vi "CC Restore Previous Setup.vi"() -> (2 "Select File":path, 3 "Restored?":bool)   [LabVIEW 2024]
panel:
  in  "Cancel":bool
  out "Contents":string
  in  "Restore":bool
  in  "Previous Setups":i32(listbox)
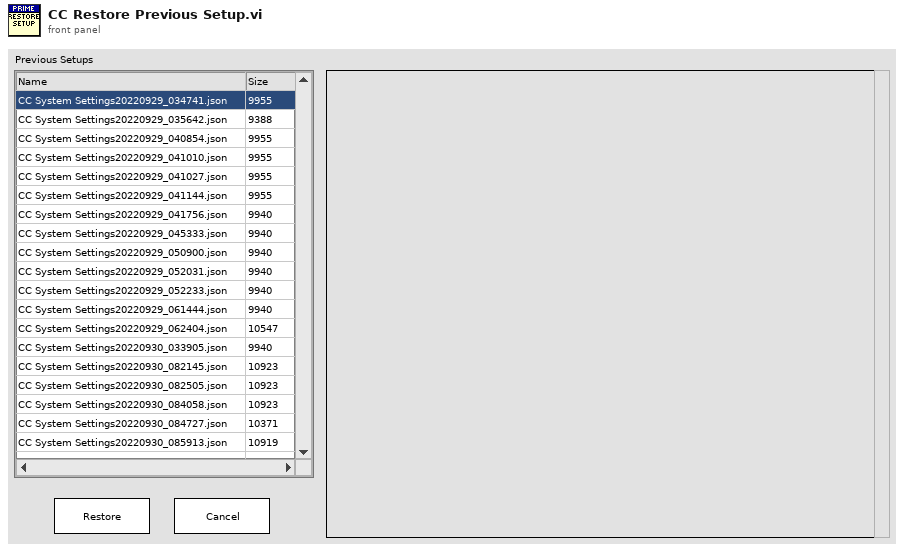
[diagram p1: front panel]
types:
  T1 = cluster{"state":refnum<user-event>, "Path":path, "Select File":path, "Restored?":bool}
  T2 = enum32{"invalid app kind", "Development System", "Run Time System", "Student Edition", "Embedded LabVIEW", "Evaluation", "Custom"}
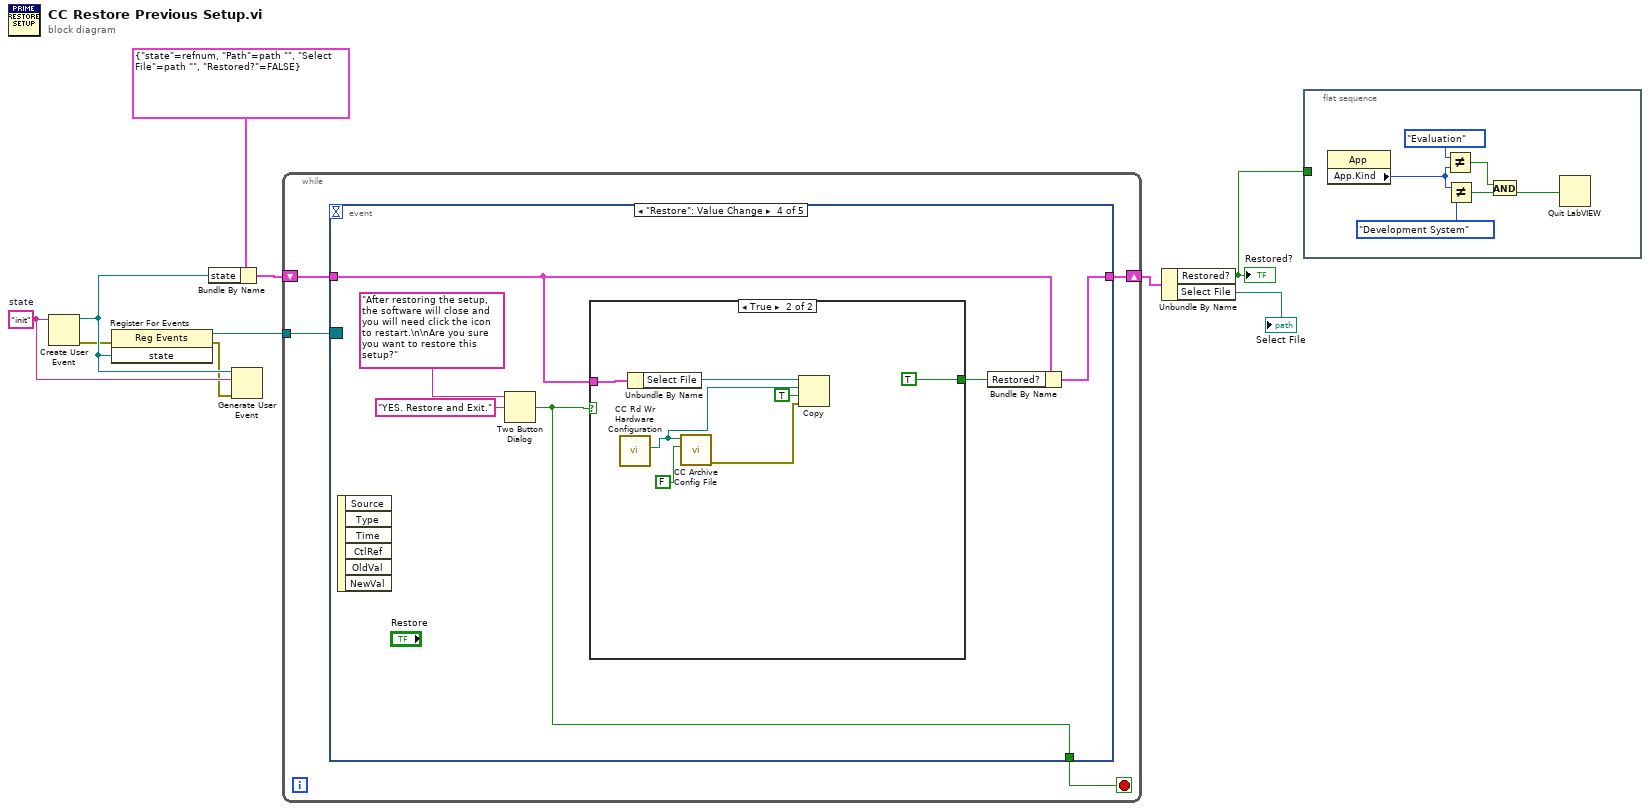
[diagram p0: block diagram]
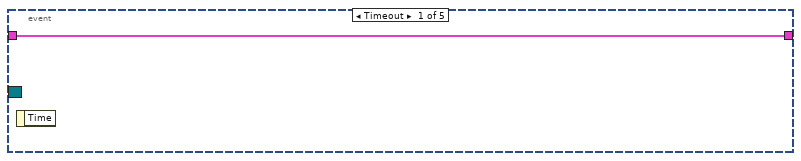
[diagram p2: hidden frame]
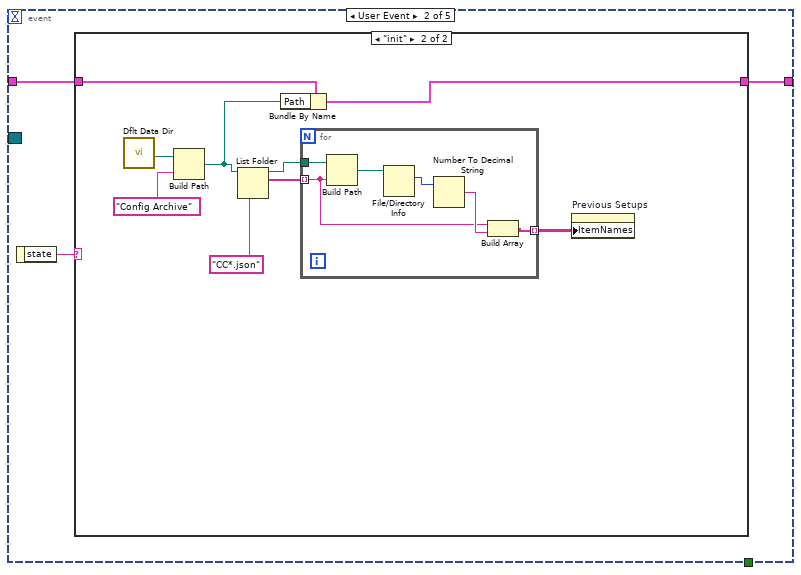
[diagram p3: hidden frame]
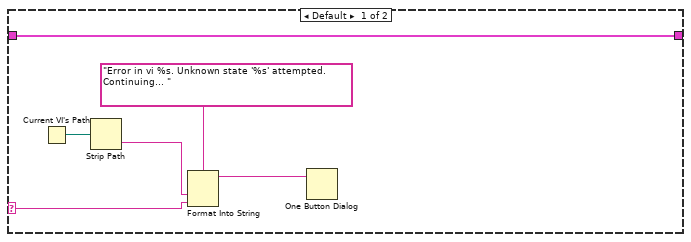
[diagram p4: hidden frame]
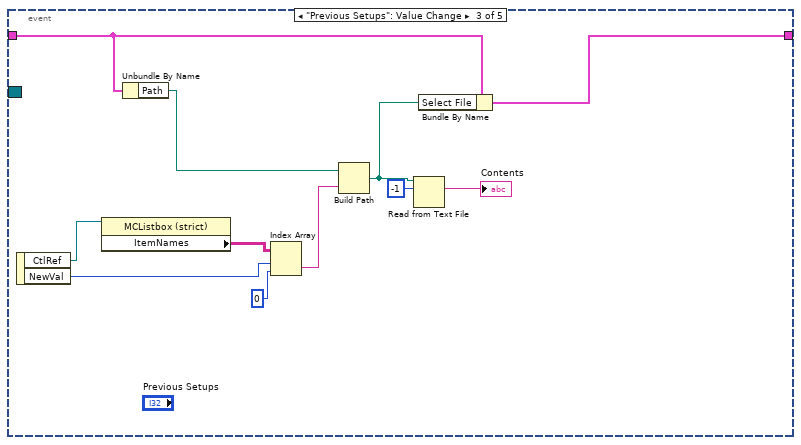
[diagram p5: hidden frame]
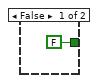
[diagram p6: hidden frame]
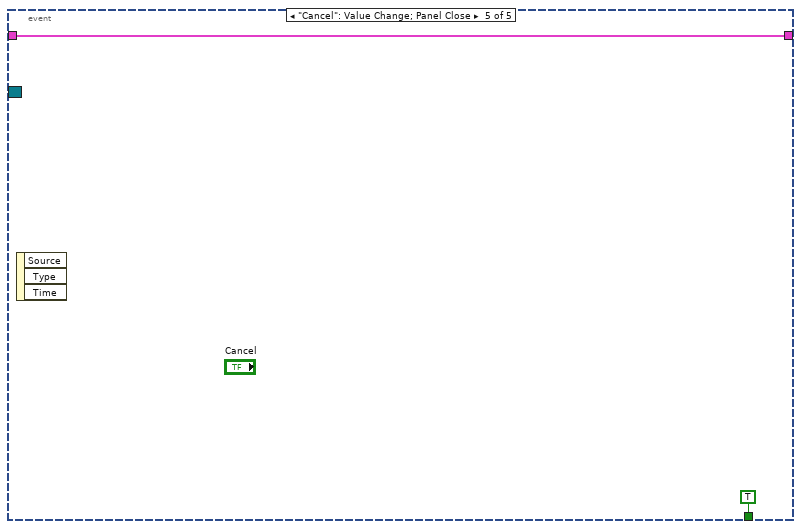
[diagram p7: hidden frame]
diagram:
  w6 = "init"  # state
  n1 = Create User Event(user event datatype=w6) -> (user event=w8:refnum<user-event>, error out=w4:errorcluster)  [unwired: 1 in]
  n2 = register-events(error in=w4, w8) -> (reference out=w7:refnum<event-registration>, error out=w5:errorcluster)  [unwired: 1 in]
  n3 = Bundle By Name(cluster=T1 {"state"=refnum, "Path"=path "", "Select File"=path "", "Restored?"=FALSE}, "state"=w8) -> (w9:T1)
  n4 = Generate User Event(user event=w8, event data cluster=w6, error in=w5) -> ()  [unwired: 1 in, 2 out]
  n5 = while {
    tunnel: w7 -> [w14]
    shift-right: [w12] -> w3
    shift-left: w9 -> [w13]
    stop <- w11 stop-if-true
    n6 = event shown="[3] \"Restore\": Value Change" {
      selector: w14 -> [_ _ _ _ _]
      dyn-events: _ -> [_ _ _ _ _]
      timeout: _ -> [_ _ _ _ _]
      tunnel: w13 -> [w15 w17 w40 w51 w66]
      tunnel: [w15 w16 w41 w52 w66] -> w12
      tunnel: [_ _ _ w54 TRUE ("Close")] -> w11
      event Timeout {
        n7 = event-data() -> ()  [unwired: 1 in, 1 out]
      }
      event User Event {
        n8 = event-data() -> ("state"=w18:string)  [unwired: 1 in]
        n9 = case shown="\"init\"" w18 {
          selector: w18 -> [w23 _]
          tunnel: w17 -> [w19 w25]
          tunnel: [w19 w26] -> w16
          frame Default {
            n10 = Current VI's Path() -> (path=w22:path)
            n11 = Strip Path(path=w22) -> (name=w21:string)  [unwired: 1 out]
            n12 = Format Into String(format string="Error in vi %s. Unknown state '%s' attempted. Continuing... ", w21, w23) -> (resulting string=w20:string)  [unwired: 2 in, 1 out]
            n13 = One Button Dialog(message=w20) -> ()  [unwired: 1 in, 1 out]
          }
          frame "init" {
            n14 = call <vilib>:"Dflt Data Dir.vi"() -> ("App:Default Data Directory"=w33:path)
            n15 = Build Path(base path=w33, name or relative path="Config Archive") -> (appended path=w27:path)
            n16 = List Folder(path=w27, pattern="CC*.json") -> (path out=w29:path, filenames=w30:string[])  [unwired: 2 in, 2 out]
            n17 = Bundle By Name(cluster=w25, "Path"=w27) -> (w26:T1)
            n18 = for {
              tunnel: w30 -> [w35] mode=indexing
              tunnel: w29 -> [w39]
              tunnel: [w34] -> w28 mode=indexing
              n19 = Build Path(base path=w39, name or relative path=w35) -> (appended path=w38:path)
              n20 = File/Directory Info(path=w38) -> (size=w37:i64)  [unwired: 1 in, 6 out]
              n21 = Number To Decimal String(number=w37) -> (decimal integer string=w36:string)  [unwired: 1 in]
              n22 = Build Array(w35, w36) -> (w34:string[])
            }
            n23 = property on="Previous Setups" class="MCListbox (strict)"("ItemNames"=w28) -> ()  [unwired: 2 in, 2 out]
          }
        }
      }
      event "Previous Setups": Value Change {
        n24 = event-data() -> ("CtlRef"=w50:refnum<vi>, "NewVal"=w48:i32)  [unwired: 1 in]
        n25 = property class="MCListbox (strict)"(reference=w50) -> ("ItemNames"=w49:string[][])  [unwired: 1 in, 2 out]
        n26 = Unbundle By Name(w40) -> ("Path"=w46:path)
        n27 = Index Array(array=w49, index (row)=w48, index (col)=0 ("disabled index (col)")) -> (element=w45:string)
        n28 = Build Path(base path=w46, name or relative path=w45) -> (appended path=w42:path)
        n29 = Read from Text File(file (use dialog)=w42, count=-1) -> (text=→"Contents":string)  [unwired: 2 in, 3 out]
        n30 = Bundle By Name(cluster=w40, "Select File"=w42) -> (w41:T1)
      }
      event "Restore": Value Change {
        n31 = event-data() -> ()  [unwired: 1 in, 6 out]
        n32 = Two Button Dialog(message="After restoring the setup, the software will close and you will need click the icon to restart.\n\nAre you sure you want to restore this setup?", 2:"YES. Restore and Exit." ("T button name (\"OK\")")) -> (T button?=w54:bool)  [unwired: 1 in]
        n33 = case shown="True" w54 {
          tunnel: w51 -> [_ w64]
          tunnel: [FALSE TRUE] -> w53
          frame False {
          }
          frame True {
            n34 = call "CC Rd Wr Hardware Configuration.vi"() -> ("File"=w61:path)  [unwired: 9 in, 2 out]
            n35 = Unbundle By Name(w64) -> ("Select File"=w62:path)
            n36 = call "CC Archive Config File.vi"("Move?"=FALSE, "config file"=w61) -> ("error out"=w59:errorcluster)  [unwired: 9 in]
            n37 = Copy(8:w59, 9:TRUE ("overwrite (F)"), 10:w61, 11:w62) -> ()  [unwired: 1 in, 3 out]
          }
        }
        n38 = Bundle By Name(cluster=w51, "Restored?"=w53) -> (w52:T1)
      }
      event "Cancel": Value Change; Panel Close {
        n39 = event-data() -> ()  [unwired: 1 in, 3 out]
      }
    }
  }
  n40 = Unbundle By Name(w3) -> ("Restored?"=w1:bool, "Select File"=→"Select File":path)
  "Restored?" <- w1
  n41 = flat-sequence {
    tunnel: w1 -> [_]
    frame #0 {
      n42 = property class="App"() -> ("App.Kind"=w67:T2)  [unwired: 2 in, 2 out]
      n43 = Not Equal?(x=T2."Evaluation" ("y"), y=w67) -> (x != y?=w68:bool)
      n44 = Not Equal?(x=w67, y=T2."Development System") -> (x != y?=w71:bool)
      n45 = And(x=w68, y=w71) -> (x .and. y?=w69:bool)
      n46 = Quit LabVIEW(quit? (T)=w69) -> ()
    }
  }
